vi "Convert to Remote Instrument State.vi"(8 "error in (no error)":errorcluster, 11 "Internal Instrument State in":T2={"Connection Info"={"VISA Resource"="", "Address"=1}, "Running"=FALSE, "Running Since"=timestamp(0 s since 1904-01-01), "Instrument State"={"Abs. Pressure"=0.0, "Amb. Pressure"=0.0, "Device"="", "Firmware Version"="", "Error Status"=FALSE, "Error Code"=0, "Error Source"="", "Gauge Pressure"=0.0, "Temperature"=0.0, "Units (0-kPa,1-PSI,2-BAR)"=0.0}} {"Instrument State"."Temperature" min=0 format="%#.2f"; "Instrument State"."Gauge Pressure" min=0 format="%#.2f"; "Instrument State"."Amb. Pressure" min=0; "Connection Info"."Address" min=1}) -> (0 "error out":errorcluster, 3 "Remote Instrument State out":variant)   [LabVIEW 2020, in "plugin_flodx_pressure.lvlib" / "plugin.lvlib" / "Instrument Manager.lvlib"]
doc: "Converts the internal instrument state cluster into the remote instrument state representation."
uses:
  Instrument Manager.lvlib
  loop/Instrument Loop State.ctl
  connection_info/Connection Info.ctl
  Instrument State.ctl
  <userlib>/RxnRover/PluginCore/src/process loops/Remote Connection Manager/ControllerScaffolds/Passive Hardware State.ctl
  <userlib>/RxnRover/PluginCore/src/RxnRover_Plugin_Core.lvlib
  <userlib>/RxnRover/PluginCore/src/process loops/Remote Connection Manager/ControllerTypes/ControllerTypes.lvlib
panel:
  out "Remote Instrument State":T1
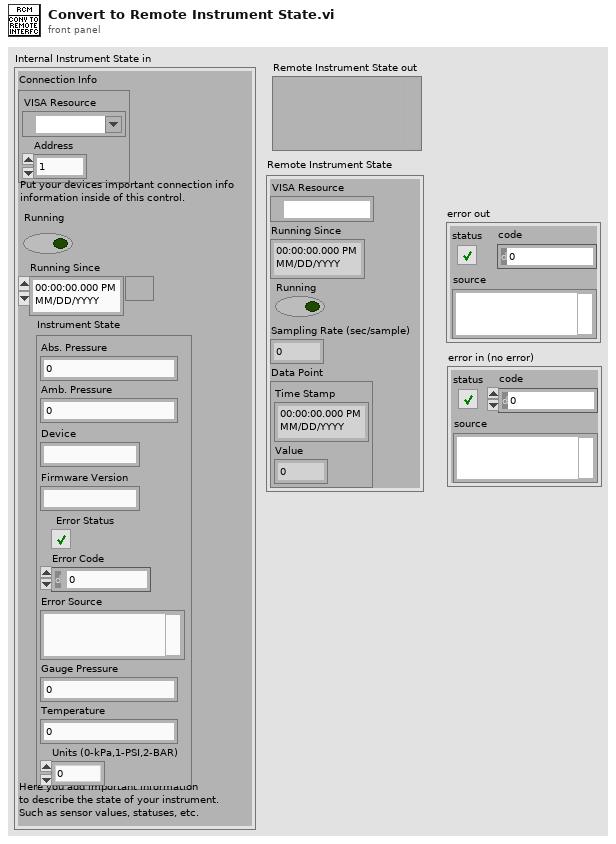
[diagram p1: front panel]
types:
  T1 = typedef "RxnRover_Plugin_Core.lvlib/Remote Connection Manager.lvlib/ControllerTypes.lvlib/Passive Hardware State.ctl" = cluster{"VISA Resource":refnum<visa-resource-name>, "Running Since":timestamp, "Running":bool, "Sampling Rate (sec/sample)":dbl, "Data Point":cluster{"Time Stamp":timestamp, "Value":dbl}}
  T2 = typedef "plugin_flodx_pressure.lvlib/plugin.lvlib/Instrument Manager.lvlib/Instrument Loop State.ctl" = cluster{"Connection Info":T3, "Running":bool, "Running Since":timestamp, "Instrument State":T4}
  T3 = typedef "plugin_flodx_pressure.lvlib/plugin.lvlib/Instrument Manager.lvlib/Connection Info.ctl" = cluster{"VISA Resource":refnum<visa-resource-name>, "Address":u8}
  T4 = typedef "plugin_flodx_pressure.lvlib/plugin.lvlib/Instrument Manager.lvlib/Instrument State.ctl" = cluster{"Abs. Pressure":sgl, "Amb. Pressure":sgl, "Device":string, "Firmware Version":string, "Error Status":bool, "Error Code":i32, "Error Source":string, "Gauge Pressure":sgl, "Temperature":sgl, "Units (0-kPa,1-PSI,2-BAR)":dbl}
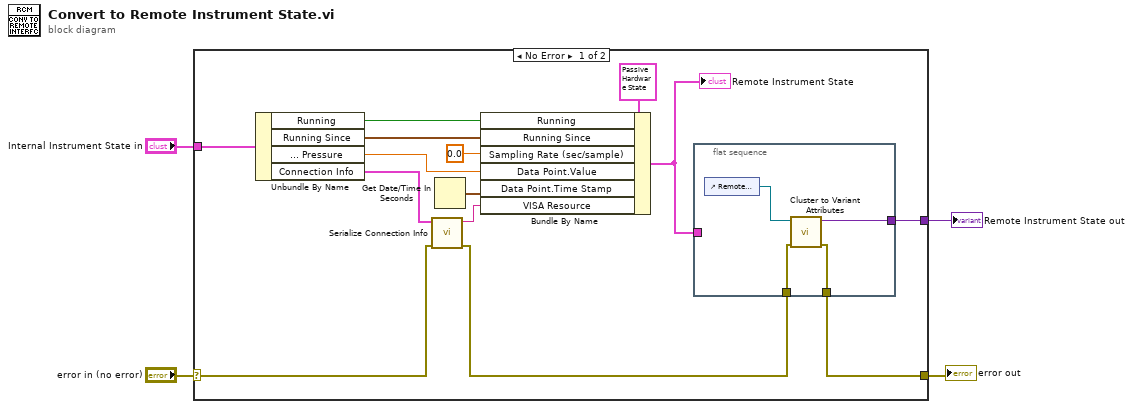
[diagram p0: block diagram]
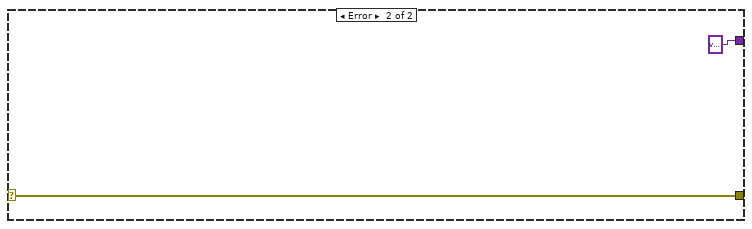
[diagram p2: hidden frame]
diagram:
  n1 = case shown="No Error" "error in (no error)" {
    selector: "error in (no error)" -> [w6 w24]
    tunnel: "Internal Instrument State in" -> [w18 _]
    tunnel: [w16 w24] -> w2
    tunnel: [w17 variant ("Variant out")] -> w1
    frame No Error {
      n2 = Unbundle By Name(w18) -> ("Running"=w15:bool, "Running Since"=w14:timestamp, "Instrument State.Abs. Pressure"=w12:sgl, "Connection Info"=w8:T3)
      n3 = call "Serialize Connection Info.vi"("error in (no error)"=w6, "Connection Info"=w8) -> ("error out 2"=w5:errorcluster, "Serialized Connection Info"=w7:string)  [unwired: 8 in]
      n4 = Get Date/Time In Seconds() -> (seconds since 1Jan1904=w11:timestamp)
      n5 = Bundle By Name(cluster=T1 {"VISA Resource"="", "Running Since"=timestamp(0 s since 1904-01-01), "Running"=FALSE, "Sampling Rate (sec/sample)"=0.0, "Data Point"={"Time Stamp"=timestamp(0 s since 1904-01-01), "Value"=0.0}} ("Instrument State"), "Running"=w15, "Running Since"=w14, "Sampling Rate (sec/sample)"=0.0, "Data Point.Value"=w12, "Data Point.Time Stamp"=w11, "VISA Resource"=w7) -> (w9:T1)
      "Remote Instrument State" <- w9
      n6 = flat-sequence {
        tunnel: [w22] -> w17
        tunnel: w5 -> [w21]
        tunnel: [w20] -> w16
        tunnel: w9 -> [_]
        frame #0 {
          n7 = control-ref of="Remote Instrument State"() -> (w19:refnum<vi>)
          n8 = call <userlib>:"Cluster to Variant Attributes.vi"("error in (no error)"=w21, "Cluster in"=w19) -> ("error out"=w20:errorcluster, "Variant out"=w22:variant)  [unwired: 8 in]
        }
      }
    }
    frame Error {
    }
  }
  "error out" <- w2
  "Remote Instrument State out" <- w1
